vi "rectanglefinder.vi"(9 "Mask":T1, 10 "Orig":T1, 11 "CameraDevRef":T2) -> (3 "Target Info":T4(array[cluster]))   [LabVIEW 2011]
uses:
  <vilib>/Rock Robotics/WPI/Camera/WPI_CameraDevRef.ctl
  <vilib>/vision/Image Controls.llb/IMAQ Image.ctl
  Program Files/National Instruments/LabVIEW 2011/examples/FRC/Vision/Rectangular Target Processing/Robot Global Data.vi
  <vilib>/vision/NI_Vision_Development_Module.lvlib
panel:
  in  "View 2":bool
  in  "Processing":enum32{"Color", "Intensity", "Intensity Open"}(tab)
  in  "Luminance":i32=255
  in  "Saturation":i32=255
  in  "Hue":i32(knob)=65 scale=0.0..255.0
  in  "Margins":cluster{"Hue":i32, "Sat":i32, "Lum":i32}={"Hue"=20, "Sat"=27, "Lum"=30} {"Sat" scale=0.0..40.0; "Lum" scale=0.0..40.0; "Hue" scale=0.0..40.0}
  in  "Range":cluster{"Lower value":sgl, "Upper value":sgl}={"Lower value"=150.0, "Upper value"=255.0} {"Lower value" scale=0.0..255.0; "Upper value" scale=0.0..255.0}
  in  "Range 2":cluster{"Lower value":sgl, "Upper value":sgl}={"Lower value"=150.0, "Upper value"=255.0} {"Lower value" scale=0.0..255.0; "Upper value" scale=0.0..255.0}
  in  "Particle Count Limit":i32=8
  in  "Area Size Limit":i32=444
  in  "Score Limits":T3={"Rect Coverage"=76.0, "Aspect Ratio"=70.0, "X Edge Strength"=40.0, "Y Edge Strength"=60.0}
  in  "Camera Type":enum16{"206", "1011"}(ring)
  in  "View":bool
  out "Original Image":T1(plugin-control)
  out "Processed Image":T1(plugin-control)
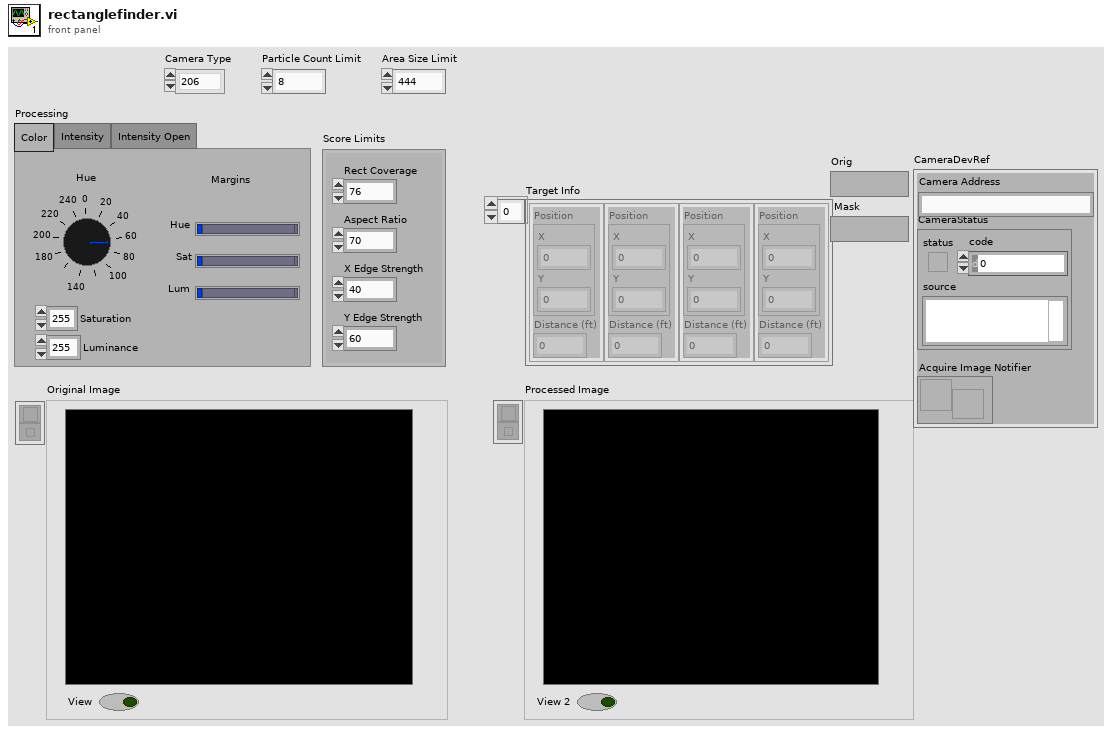
[diagram p1: front panel]
types:
  T1 = typedef "IMAQ Image.ctl" = refnum<image>
  T2 = typedef "WPI_CameraDevRef.ctl" = cluster{"Camera Address":string, "CameraStatus":errorcluster, "Acquire Image Notifier":refnum<notifier>}
  T3 = cluster{"Rect Coverage":dbl, "Aspect Ratio":dbl, "X Edge Strength":dbl, "Y Edge Strength":dbl}
  T4 = cluster{"Position":cluster{"X":dbl, "Y":dbl}, "Distance (ft)":dbl}[]
  T5 = typedef "WPI_CameraImageSize.ctl" = enum16{"640x480", "320x240", "160x120"}
  T6 = enum32{"AutoM", "Close", "Dilate", "Erode", "Gradient", "Gradient out", "Gradient in", "Hit miss", "Open", "PClose", "POpen", "Thick", "Thin"}
  T7 = cluster{cluster{"Left":dbl, "Top":dbl, "Right":dbl, "Bottom":dbl}, dbl[]}[]
  T8 = cluster{"Left":dbl, "Top":dbl, "Right":dbl, "Bottom":dbl}
  T9 = cluster{"Target Center (-1 to 1)":cluster{"X":dbl, "Y":dbl}, "Distance (ft)":dbl}
  T10 = cluster{"Target Center (-1 to 1)":cluster{"X":dbl, "Y":dbl}, "Distance (ft)":dbl}[]
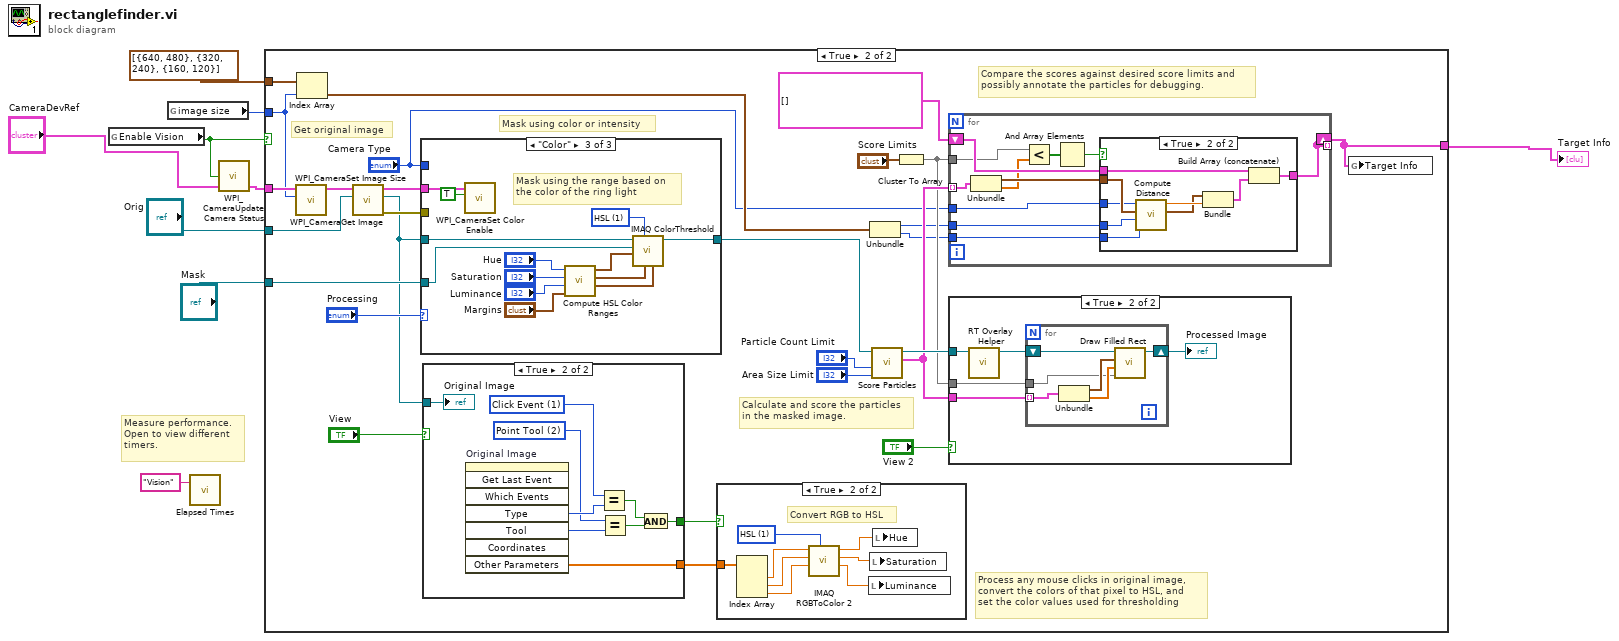
[diagram p0: block diagram]
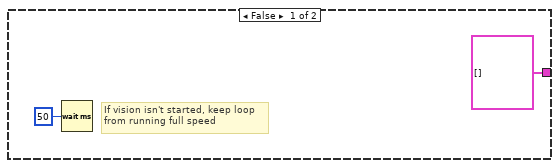
[diagram p2: hidden frame]
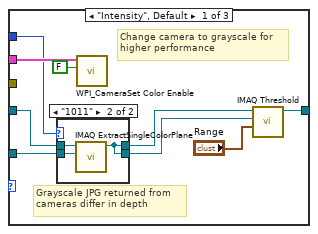
[diagram p4: hidden frame]
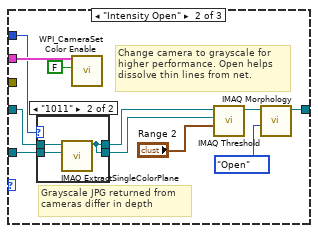
[diagram p6: hidden frame]
diagram:
  # "Measure performance.\nOpen to view different\ntimers."
  n1 = global read "Robot Global Data.vi" "Enable Vision"() -> (w7:bool)
  n2 = global read "Robot Global Data.vi" "image size"() -> (w5:T5)
  n3 = call "Elapsed Times.vi"("Call Name"="Vision") -> ()  [unwired: 2 in, 1 out]
  n4 = call <vilib>:"WPI_CameraUpdate Camera Status.vi"("CameraDevRef In"="CameraDevRef", "Enable Vision"=w7) -> ("CameraDevRef Out"=w8:T2)  [unwired: 3 in]
  n5 = case shown="True" w7 {
    tunnel: "Orig" -> [_ w29]
    tunnel: w8 -> [_ w25]
    tunnel: w5 -> [_ w20]
    tunnel: "Mask" -> [_ w15]
    tunnel: cluster{i32, i32}[] [{640, 480}, {320, 240}, {160, 120}] -> [_ w19]
    tunnel: [T4 [] w12] -> w9
    frame False {
      # "If vision isn't started, keep loop\nfrom running full speed"
      n6 = Wait (ms)(milliseconds to wait=u32 50) -> ()  [unwired: 1 out]
    }
    frame True {
      # "Compare the scores against desired score limits and\npossibly annotate the particles for debugging."
      # "Process any mouse clicks in original image,\nconvert the colors of that pixel to HSL, and\nset the color values used for thresholding"
      # "Calculate and score the particles\nin the masked image."
      # "Mask using color or intensity"
      # "Get original image"
      n7 = call <vilib>:"WPI_CameraSet Image Size.vi"("Image Size"=w20, "CameraDevRef"=w25) -> ("CameraDevRef Out"=w26:T2)  [unwired: 8 in, 1 out]
      n8 = Index Array(array=w19, index=w20) -> (element=w16:cluster{i32, i32})
      n9 = call <vilib>:"WPI_CameraGet Image.vi"("Image"=w29, "CameraDevRef"=w26) -> ("error out"=w27:errorcluster, "Image Out"=w14:T1, "CameraDevRef Out"=w28:T2)  [unwired: 7 in]
      n10 = case shown="\"Color\"" "Processing" {
        tunnel: w14 -> [w51 w63 w89]
        tunnel: [w54 w68 w88] -> w23
        tunnel: w28 -> [w52 w66 w79]
        tunnel: w27 -> [_ _ _]
        tunnel: w15 -> [w50 w64 w77]
        tunnel: "Camera Type" -> [w49 w65 _]
        frame "Intensity", Default {
          # "Grayscale JPG returned from\ncameras differ in depth"
          # "Change camera to grayscale for\nhigher performance"
          n11 = case shown="\"1011\"" w49 {
            tunnel: w51 -> [w57 w60]
            tunnel: w50 -> [w56 w59]
            tunnel: [w57 w58] -> w48
            tunnel: [w56 w58] -> w47
            frame "206", Default {
            }
            frame "1011" {
              n12 = call "IMAQ ExtractSingleColorPlane"("Image Dst"=w59, "Image Src"=w60) -> ("Image Dst Out"=w58:T1)  [unwired: 8 in, 1 out]
            }
          }
          n13 = call <vilib>:"WPI_CameraSet Color Enable.vi"("Color Enabled"=FALSE, "CameraDevRef"=w52) -> ()  [unwired: 8 in, 2 out]
          n14 = call "IMAQ Threshold"("Range"="Range", "Image Dst"=w47, "Image Src"=w48) -> ("Image Dst Out"=w54:T1)  [unwired: 3 in, 5 out]
        }
        frame "Intensity Open" {
          # "Grayscale JPG returned from\ncameras differ in depth"
          # "Change camera to grayscale for\nhigher performance. Open helps\ndissolve thin lines from net."
          n15 = case shown="\"1011\"" w65 {
            tunnel: w63 -> [w73 w76]
            tunnel: w64 -> [w72 w75]
            tunnel: [w73 w74] -> w62
            tunnel: [w72 w74] -> w61
            frame "206", Default {
            }
            frame "1011" {
              n16 = call "IMAQ ExtractSingleColorPlane"("Image Dst"=w75, "Image Src"=w76) -> ("Image Dst Out"=w74:T1)  [unwired: 8 in, 1 out]
            }
          }
          n17 = call <vilib>:"WPI_CameraSet Color Enable.vi"("Color Enabled"=FALSE, "CameraDevRef"=w66) -> ()  [unwired: 8 in, 2 out]
          n18 = call "IMAQ Threshold"("Range"="Range 2", "Image Dst"=w61, "Image Src"=w62) -> ("Image Dst Out"=w69:T1)  [unwired: 3 in, 5 out]
          n19 = call "IMAQ Morphology"("Operation"=T6."Open", "Image Src"=w69) -> ("Image Dst Out"=w68:T1)  [unwired: 8 in, 1 out]
        }
        frame "Color" {
          w87 = u16 1 items=["RGB", "HSL", "HSV", "HSI"] ("Color Mode")
          # "Mask using the range based on\nthe color of the ring light"
          n20 = call <vilib>:"WPI_CameraSet Color Enable.vi"("Color Enabled"=TRUE, "CameraDevRef"=w79) -> ()  [unwired: 8 in, 2 out]
          n21 = call "Compute HSL Color Ranges.vi"("Margins"="Margins", "Luminance"="Luminance", "Saturation"="Saturation", "Hue"="Hue") -> ("Lum Range"=w84:cluster{i32, i32}, "Sat Range"=w85:cluster{i32, i32}, "Hue Range"=w86:cluster{i32, i32})  [unwired: 5 in]
          n22 = call "IMAQ ColorThreshold"("Blue or Luma or Val or Inten Range"=w84, "Green or Sat Range"=w85, "Color Mode"=w87, "Red or Hue Range"=w86, "Image Dst"=w77, "Image Src"=w89) -> ("Image Dst Out"=w88:T1)  [unwired: 4 in, 1 out]
        }
      }
      n23 = case shown="True" "View" {
        tunnel: w14 -> [_ w109]
        tunnel: [_ w104] -> w22
        tunnel: [_ w101] -> w21
        frame False {
        }
        frame True {
          w102 = 2 items=["None", "Selection Tool", "Point Tool", "Line Tool", "Rectangle Tool", "Oval Tool", "Polygon Tool", "ClosedFreehandTool", "Annulus Tool", "Rotated Rectangle Tool", "Zoom Tool", "Pan Tool", "Polyline Tool", "Freehand Tool"] ("Tool")
          w103 = 1 items=["No Event"=0, "Click Event"=1, "Draw Event"=2, "Size Event"=4, "Scroll Event"=5, "Double Click Event"=8] ("Type")
          n24 = invoke on="Original Image" class="ImageControl" method="Get Last Event"() -> ("Type"=w105:i32, "Tool"=w108:i32, "Other Parameters"=w101:sgl[])  [unwired: 8 in, 5 out]
          n25 = Equal?(x=w103, y=w105) -> (x = y?=w106:bool)
          n26 = Equal?(x=w102, y=w108) -> (x = y?=w107:bool)
          n27 = And(x=w106, y=w107) -> (x .and. y?=w104:bool)
          "Original Image" <- w109
        }
      }
      n28 = case shown="True" w22 {
        tunnel: w21 -> [_ w46]
        frame False {
        }
        frame True {
          w45 = u16 1 items=["RGB", "HSL", "HSV", "HSI", "CIE L*a*b*", "CIE XYZ"] ("Color Mode")
          # "Convert RGB to HSL"
          n29 = Index Array(array=w46) -> (element #1=w44:sgl, element #2=w42:sgl, element #3=w40:sgl)  [unwired: 3 in]
          n30 = call "IMAQ RGBToColor 2"("Color Mode"=w45, "Blue value"=w40, "Green value"=w42, "Red value"=w44) -> ("Blue or Luma or Val or Inten or Z or b*value"=w39:dbl, "Green or Sat or Y or a* value"=w41:dbl, "Red or Hue or X or L* value"=w43:dbl)  [unwired: 4 in, 1 out]
          n31 = local write "Luminance"(w39) -> ()
          n32 = local write "Saturation"(w41) -> ()
          n33 = local write "Hue"(w43) -> ()
        }
      }
      n34 = Unbundle(w16) -> (w18:i32, w17:i32)
      n35 = call "Score Particles.vi"("Area Size Limit"="Area Size Limit", "Particle Count Limit"="Particle Count Limit", "Image Refnum in"=w23) -> ("Scored Particle Info"=w34:T7, "Image Refnum out"=w37:T1)  [unwired: 7 in]
      n36 = Cluster To Array(cluster="Score Limits") -> (array=w32:dbl[])
      n37 = for {
        shift-right: [w110] -> w12
        shift-left: T4 [] -> [w120]
        tunnel: w18 -> [w119]
        tunnel: w34 -> [w117] mode=indexing
        tunnel: w32 -> [w112]
        tunnel: "Camera Type" -> [w116]
        tunnel: w17 -> [w111]
        tunnel: [w110] -> _ mode=indexing
        n38 = Unbundle(w117) -> (w118:T8, w113:dbl[])
        n39 = Less?(x=w112, y=w113) -> (x < y?=w115:bool[])
        n40 = And Array Elements(Boolean array=w115) -> (logical AND=w114:bool)
        n41 = case shown="True" w114 {
          tunnel: w120 -> [w121 w130]
          tunnel: [w121 w129] -> w110
          tunnel: w118 -> [_ w125]
          tunnel: w119 -> [_ w127]
          tunnel: w116 -> [_ w124]
          tunnel: w111 -> [_ w123]
          frame False {
          }
          frame True {
            n42 = call "Compute Distance.vi"("Y Image Resolution"=w123, "X Image Resolution"=w127, "Bounding Box"=w125, "Camera Type"=w124) -> ("Target Center (-1 to 1)"=w122:cluster{"X":dbl, "Y":dbl}, "Distance (ft)"=w126:dbl)  [unwired: 6 in]
            n43 = Bundle("Target Center (-1 to 1)"=w122, "Distance (ft)"=w126) -> (w128:T9)  [unwired: 1 in]
            n44 = Build Array (concatenate)(w130, w128) -> (w129:T10)
          }
        }
      }
      n45 = case shown="True" "View 2" {
        tunnel: w37 -> [_ w91]
        tunnel: w34 -> [_ w93]
        tunnel: w32 -> [_ w92]
        frame False {
        }
        frame True {
          n46 = call "RT Overlay Helper.vi"("Refnum in"=w91) -> ("Refnum out"=w94:T1)  [unwired: 10 in]
          n47 = for {
            shift-right: [w99] -> w90
            shift-left: w94 -> [w100]
            tunnel: w93 -> [w96] mode=indexing
            tunnel: w92 -> [w95]
            n48 = Unbundle(w96) -> (w97:T8, w98:dbl[])
            n49 = call "Draw Filled Rect.vi"("Limits"=w95, "Scores"=w98, "Bounding Box"=w97, "image in"=w100) -> ("image out"=w99:T1)  [unwired: 7 in]
          }
          "Processed Image" <- w90
        }
      }
      n50 = global write "Robot Global Data.vi" "Target Info"(w12) -> ()
    }
  }
  "Target Info" <- w9
